vi "get_pair_Pump_state.vi"(8 "Error In":errorcluster, 10 "Система in":T1={"Давление заданное"=0.3, "Давление в системе"=100.0, "Расход заданый"=0.0, "Расход текущий"=99.99, "Объём заданный"=0.0, "Объём текущий"=0.0, "Старт давление"=FALSE, "Старт расход"=FALSE, "Сброс объёма"=FALSE, "plc_control"=FALSE, "lag_control"=FALSE, "mstop_control"=FALSE, "Давление"={"АЦП CH 0"=0.0, "АЦП CH 1"=0.0, "АЦП CH 2"=0.0, "АЦП CH 3"=0.0, "АЦП CH 4"=0.0, "АЦП CH 5"=0.0, "АЦП CH 6"=0.0, "АЦП CH 7"=0.0}, "Modbus"={"Массив чтения"=[], "Массив записи"=[]}} {"Давление"."АЦП CH 7" format="%.3f"; "Давление"."АЦП CH 6" format="%.3f"; "Давление"."АЦП CH 5" format="%.3f"; "Давление"."АЦП CH 4" format="%.3f"; "Давление"."АЦП CH 3" format="%.3f"; "Давление"."АЦП CH 2" format="%.3f"; "Давление"."АЦП CH 1" format="%.3f"; "Давление"."АЦП CH 0" format="%.3f"; "Объём текущий" min=0.0 max=9999.0 step=0.0001 format="%#_5f"; "Объём заданный" min=0.0 max=9999.0 step=0.0001 format="%#_5f"; "Расход текущий" format="%#_5f"; "Расход заданый" min=0.0 max=40.0 step=0.0001 format="%#_5f"; "Давление в системе" format="%.3f"; "Давление заданное" min=0.3 max=100.0 step=0.01 format="%#_5f"}, 11 "queue_Pair in":refnum<queue>) -> (0 "Error Out":errorcluster, 3 "queue_Pair out":refnum<queue>)   [LabVIEW 2023, in "pump_Lib.lvlib"]
uses:
  pump_Lib.lvlib
  TypeDef/pair_Type.ctl
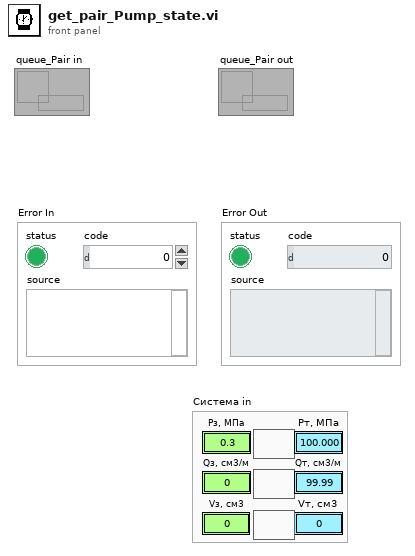
[diagram p1: front panel]
types:
  T1 = typedef "pump_Lib.lvlib/pair_Type.ctl" = cluster{"Давление заданное":dbl, "Давление в системе":dbl, "Расход заданый":dbl, "Расход текущий":dbl, "Объём заданный":dbl, "Объём текущий":dbl, "Старт давление":bool, "Старт расход":bool, "Сброс объёма":bool, "plc_control":bool, "lag_control":bool, "mstop_control":bool, "Давление":cluster{"АЦП CH 0":dbl, "АЦП CH 1":dbl, "АЦП CH 2":dbl, "АЦП CH 3":dbl, "АЦП CH 4":dbl, "АЦП CH 5":dbl, "АЦП CH 6":dbl, "АЦП CH 7":dbl}, "Modbus":cluster{"Массив чтения":u16[], "Массив записи":u16[]}}
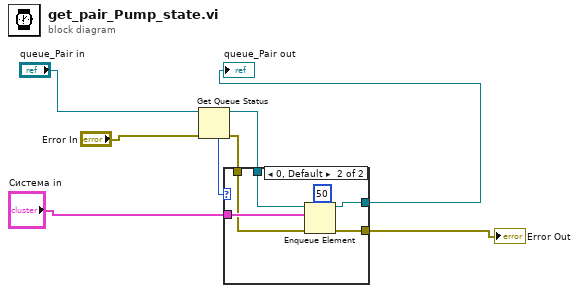
[diagram p0: block diagram]
diagram:
  n1 = Get Queue Status(queue="queue_Pair in", error in (no error)="Error In") -> (queue out=w7:refnum<queue>, error out=w6:errorcluster, # elements in queue=w4:i32)  [unwired: 1 in, 5 out]
  n2 = case shown="0, Default" w4 {
    tunnel: w7 -> [w10 w15]
    tunnel: [w10 w14] -> w2
    tunnel: "Система in" -> [_ w13]
    tunnel: w6 -> [w9 w12]
    tunnel: [w9 w11] -> w5
    frame 1 {
    }
    frame 0, Default {
      n3 = Enqueue Element(queue=w15, element=w13, timeout in ms (-1)=50, error in (no error)=w12) -> (queue out=w14:refnum<queue>, error out=w11:errorcluster)  [unwired: 1 out]
    }
  }
  "Error Out" <- w5
  "queue_Pair out" <- w2
